vi "pH_所有参数读取.vi"(8 "error in (no error)":errorcluster caption="错误输入（无错误）", 11 "MB session in":refnum<class "MB_Master.lvclass">) -> (0 "error out":errorcluster caption="错误输出", 2 "输出值":T1 {"电极型号标志" items=["NULL", "pH", "Cond", "DO", "Turb"]; "电极状态标志" items=["OK", "第一点校正通过", "第二点校正通过", "校正失败,电极零点超出范围", "校正失败,电极斜率超出范围", "第三点校正通过"]}, 3 "MB session out":refnum<class "MB_Master.lvclass">)   [LabVIEW 2016, in "斯坦道多参数.lvlib"]
uses:
  <vilib>/Plasmionique/MB Master/MB_Master/MB_Master.lvclass
  <vilib>/Plasmionique/MB Master/MB Master.lvlib
  <vilib>/ptbypt/NI_PtbyPt.lvlib
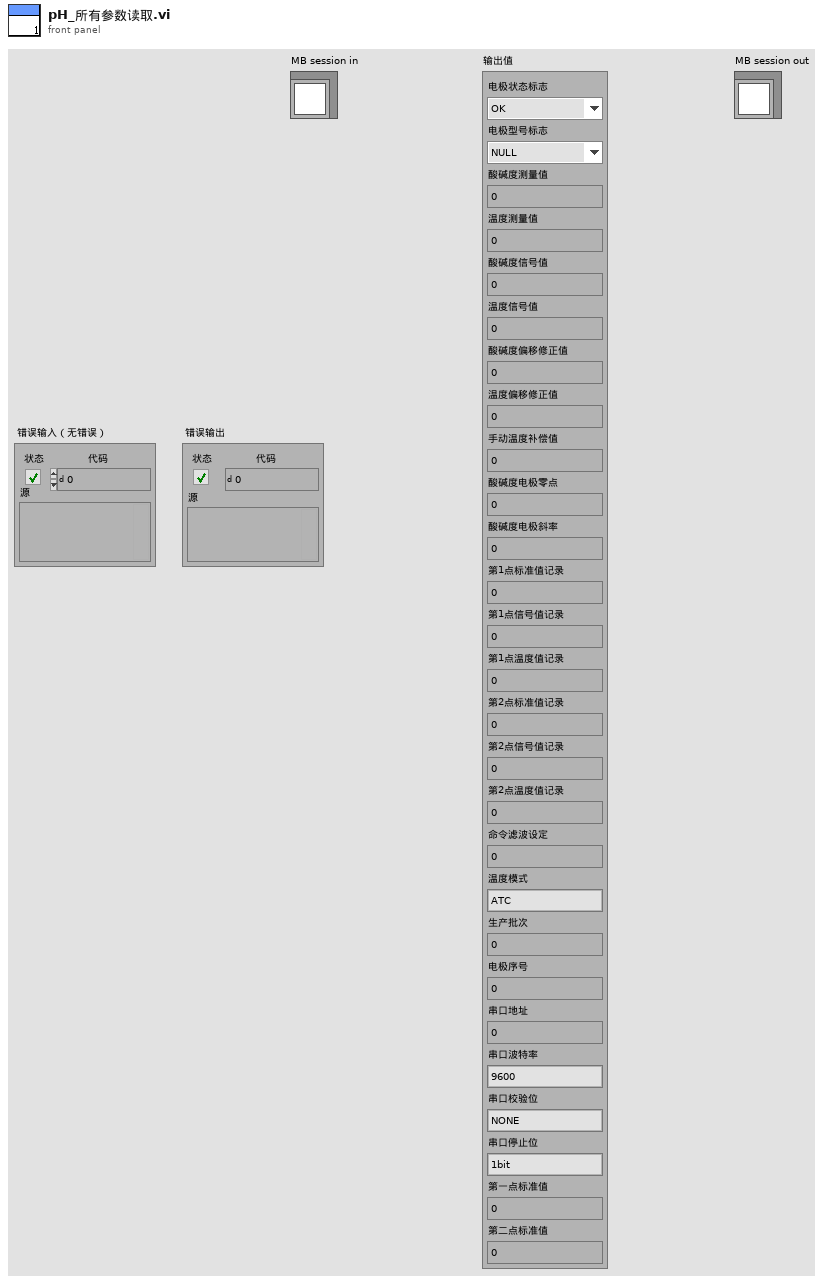
[diagram p1: front panel]
types:
  T1 = cluster{"电极状态标志":u16, "电极型号标志":u16, "酸碱度测量值":sgl, "温度测量值":sgl, "酸碱度信号值":sgl, "温度信号值":sgl, "酸碱度偏移修正值":sgl, "温度偏移修正值":sgl, "手动温度补偿值":sgl, "酸碱度电极零点":sgl, "酸碱度电极斜率":sgl, "第1点标准值记录":sgl, "第1点信号值记录":sgl, "第1点温度值记录":sgl, "第2点标准值记录":sgl, "第2点信号值记录":sgl, "第2点温度值记录":sgl, "命令滤波设定":u16, "温度模式":enum16{"ATC", "MTC"}, "生产批次":u16, "电极序号":u16, "串口地址":u16, "串口波特率":enum16{"9600", "19200", "115200"}, "串口校验位":enum16{"NONE", "ODD", "EVEN"}, "串口停止位":enum16{"1bit", "2bit"}, "第一点标准值":sgl, "第二点标准值":sgl}
  T2 = cluster{u16, u16, "Filtered x":dbl, "数值":sgl, "数值":sgl, "数值":sgl, "数值":sgl, "数值":sgl, "数值":sgl, "数值":sgl, "数值":sgl, "数值":sgl, "数值":sgl, "数值":sgl, "数值":sgl, "数值":sgl, "数值":sgl, u16, u16, u16, u16, u16, u16, u16, u16, "数值":sgl, "数值":sgl}
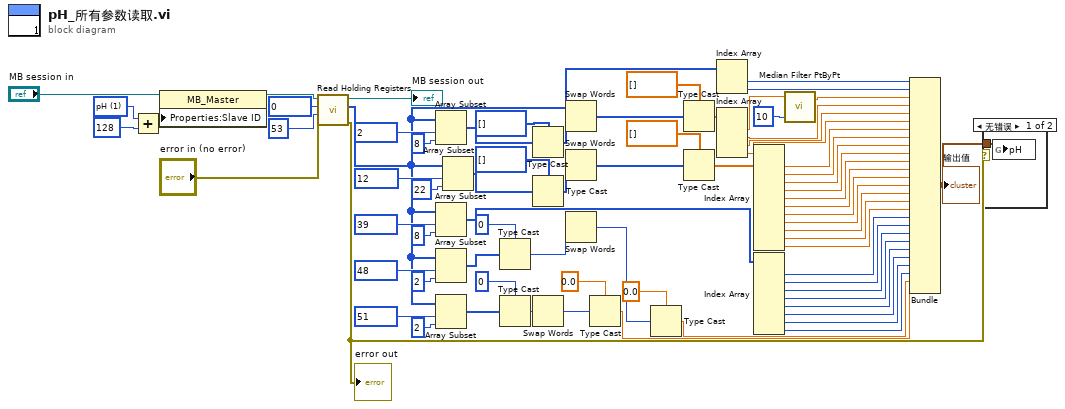
[diagram p0: block diagram]
diagram:
  w74 = u16 1 items=["NULL", "pH", "Cond", "DO", "Turb"] ("数值")
  n1 = Add(x=w74, y=u16 128) -> (x+y=w73:u16)
  n2 = property class="MB_Master"(reference="MB session in", "Properties:Slave ID"=w73) -> (reference out=w8:refnum<class "MB_Master.lvclass">)  [unwired: 1 in, 1 out]
  n3 = call <vilib>:"Read Holding Registers.vi"("error in (no error)"="error in (no error)", "quantity"=u16 53, "starting address"=u16 0, "MB session in"=w8) -> ("error out"=w7:errorcluster, "Registers"=w22:u16[], "MB session out"=→"MB session out":refnum<class "MB_Master.lvclass">)  [unwired: 5 in]
  "error out" <- w7
  n4 = Array Subset(array=w22, index=u16 2 ("starting address"), length=8 ("长度")) -> (w62:u16[])
  n5 = Array Subset(array=w22, index=u16 39 ("starting address"), length=8 ("长度")) -> (w35:u16[])
  n6 = Array Subset(array=w22, index=u16 48 ("starting address"), length=2 ("长度")) -> (w17:u16[])
  n7 = Array Subset(array=w22, index=u16 51 ("starting address"), length=2 ("长度")) -> (w12:u16[])
  n8 = Array Subset(array=w22, index=u16 12 ("starting address"), length=22 ("长度")) -> (w52:u16[])
  n9 = Type Cast(type=u32 0 ("数值"), x=w17) -> (*(type *) &x=w20:u32)
  n10 = Type Cast(type=u32 0 ("数值"), x=w12) -> (*(type *) &x=w14:u32)
  n11 = Type Cast(type=u32[] [] ("数组 2"), x=w62) -> (*(type *) &x=w64:u32[])
  n12 = Type Cast(type=u32[] [] ("数组 2"), x=w52) -> (*(type *) &x=w55:u32[])
  n13 = Swap Words(1:w14) -> (0:w13:u32)
  n14 = Swap Words(1:w64) -> (0:w66:u32[])
  n15 = Swap Words(1:w55) -> (0:w56:u32[])
  n16 = Swap Words(1:w20) -> (0:w21:u32)
  n17 = Type Cast(type=sgl 0.0 ("数值"), x=w13) -> (*(type *) &x=w10:sgl)
  n18 = Type Cast(type=sgl 0.0 ("数值"), x=w21) -> (*(type *) &x=w11:sgl)
  n19 = Type Cast(type=sgl[] [] ("数组 2"), x=w66) -> (*(type *) &x=w61:sgl[])
  n20 = Type Cast(type=sgl[] [] ("数组 2"), x=w56) -> (*(type *) &x=w51:sgl[])
  n21 = Index Array(array=w22) -> (element #1=w69:u16, element #2=w68:u16)  [unwired: 2 in]
  n22 = Index Array(array=w61) -> (element #1=w2:sgl, element #2=w60:sgl, element #3=w59:sgl, element #4=w58:sgl)  [unwired: 4 in]
  n23 = Index Array(array=w51) -> (element #1=w50:sgl, element #2=w49:sgl, element #3=w48:sgl, element #4=w47:sgl, element #5=w46:sgl, element #6=w45:sgl, element #7=w44:sgl, element #8=w43:sgl, element #9=w42:sgl, element #10=w41:sgl, element #11=w40:sgl)  [unwired: 11 in]
  n24 = Index Array(array=w35) -> (element #1=w34:u16, element #2=w33:u16, element #3=w32:u16, element #4=w31:u16, element #5=w30:u16, element #6=w29:u16, element #7=w28:u16, element #8=w27:u16)  [unwired: 8 in]
  n25 = call <vilib>:"Median Filter PtByPt.vi"("rank"=10, "x"=w2) -> ("Filtered x"=w1:dbl)  [unwired: 2 in, 1 out]
  n26 = Bundle(w69, w68, "Filtered x"=w1, "数值"=w60, "数值"=w59, "数值"=w58, "数值"=w50, "数值"=w49, "数值"=w48, "数值"=w47, "数值"=w46, "数值"=w45, "数值"=w44, "数值"=w43, "数值"=w42, "数值"=w41, "数值"=w40, w34, w33, w32, w31, w30, w29, w28, w27, "数值"=w11, "数值"=w10) -> (w6:T2)  [unwired: 1 in]
  "输出值" <- w6
  n27 = case shown="无错误" w7 {
    tunnel: w6 -> [w75 _]
    frame No Error {
      n28 = global write "国弘过程全局变量.vi" "pH"(w75) -> ()
    }
    frame Error {
    }
  }
